vi "To String.vi"(8 "error in (no error)":errorcluster, 11 "Double Float in":refnum<class "Abs_Double Float 1D.lvclass">) -> (0 "error out":errorcluster, 2 "String":string, 3 "Double Float out":refnum<class "Abs_Double Float 1D.lvclass">)   [LabVIEW 2021, in "Abs_Double Float 1D.lvclass"]
uses:
  Abs_Double Float 1D.lvclass
  C:/TSA/LV_Abstract/Source/Abs_Types/Array/Abs_Array.lvclass
  C:/TSA/LV_Abstract/Source/Abs_Types/Numeric 1D/Abs_Numeric_1D.lvclass
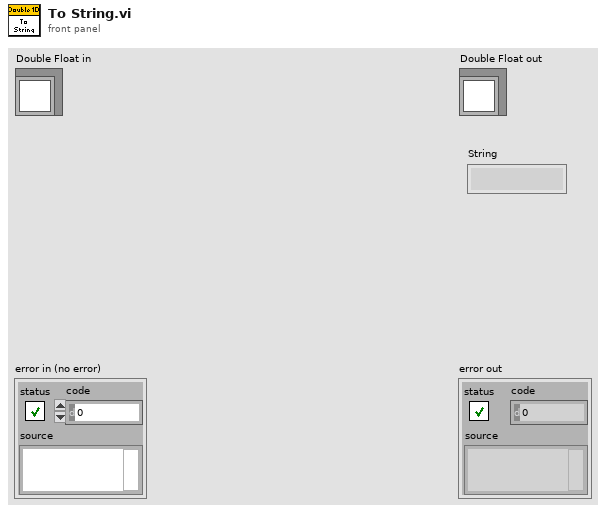
[diagram p1: front panel]
types:
  T1 = typedef "Abs_Double Float 1D.lvclass/Type.ctl" = dbl[]
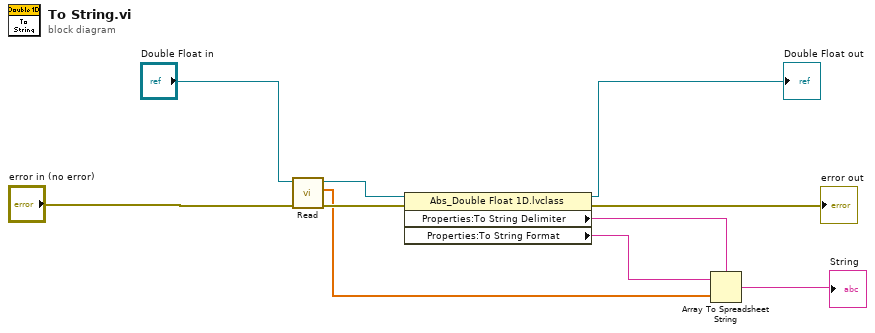
[diagram p0: block diagram]
diagram:
  n1 = call-dynamic "Read.vi"("error in (no error)"="error in (no error)", "Double Float.lvclass_340760 in"="Double Float in") -> ("error out"=w7:errorcluster, "Value"=w6:T1, "Double Float.lvclass_340760 out"=w8:refnum<class "Abs_Double Float 1D.lvclass">)  [unwired: 7 in]
  n2 = property class="Abs_Double Float 1D.lvclass"(reference=w8, error in=w7) -> (reference out=→"Double Float out":refnum<class "Abs_Double Float 1D.lvclass">, error out=→"error out":errorcluster, "Properties:To String Delimiter"=w1:string, "Properties:To String Format"=w5:string)
  n3 = Array To Spreadsheet String(delimiter (Tab)=w1, array=w6, 3:w5) -> (spreadsheet string=→"String":string)
